vi "Get XML Custom Device Version.vi"(8 "error in (no error)":errorcluster, 11 "Device Ref in":T1 format="%.0x") -> (0 "error out":errorcluster, 2 "Version":string, 3 "Device Ref out":T1 format="%.0x")   [LabVIEW 2027, in "System Monitor System Explorer.lvlib"]
uses:
  System Monitor System Explorer.lvlib
  C:/NetCore/niveristand-system-monitor-custom-device/Source/System Explorer/Get XML Custom Device Version.vi/NationalInstruments.VeriStand.SystemDefinitionAPI
  NationalInstruments.VeriStand.SystemDefinitionAPI
  <vilib>/NI VeriStand/Custom Device API/Custom Device API.lvlib
  <vilib>/NI VeriStand/Custom Device API/Custom Device Item Ref.ctl
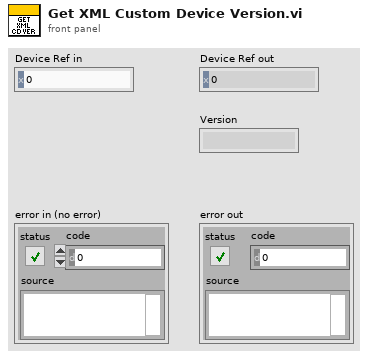
[diagram p1: front panel]
types:
  T1 = typedef "Custom Device API.lvlib/Custom Device Item Ref.ctl" = u64
  T2 = typedef "Custom Device API.lvlib/Custom Device Item Info.ctl" = cluster{"Name":string, "Is Channel":bool, "GUID":string, "Is Waveform":bool}
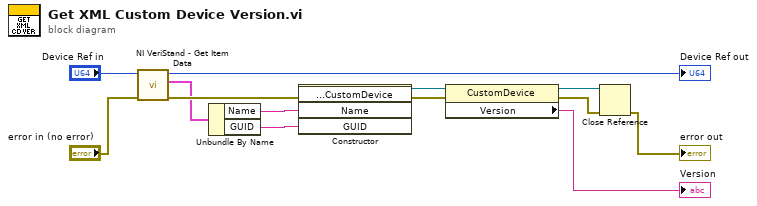
[diagram p0: block diagram]
diagram:
  n1 = call <vilib>:"NI VeriStand - Get Item Data.vi"("error in (no error)"="error in (no error)", "Item Ref in"="Device Ref in") -> ("error out"=w8:errorcluster, "Item Info"=w5:T2, "Item Ref out"=→"Device Ref out":T1)  [unwired: 6 in, 1 out]
  n2 = Unbundle By Name(w5) -> ("Name"=w6:string, "GUID"=w7:string)
  n3 = constructor class="CustomDevice"(error in=w8, "Name"=w6, "GUID"=w7) -> (reference out=w10:refnum<k39>, error out=w9:errorcluster)  [unwired: 2 in, 3 out]
  n4 = property class="CustomDevice"(reference=w10, error in=w9) -> (reference out=w12:refnum<k39>, error out=w11:errorcluster, "Version"=→"Version":string)
  n5 = Close Reference(reference=w12, error in (no error)=w11) -> (error out=→"error out":errorcluster)
